vi "CreateFixedLengthString.vi"(10 "RequiredStringLength":i32, 11 "StringIn":string) -> (2 "ByteArray":u8[](array[numeric]), 3 "DLLString":string)   [LabVIEW 2023]
doc: "Use this convenience VI when providing a string of a certain length (filled with NULL) is required. Typically when writing a SDT-file.\n\ninfo@becker-hickl.com"
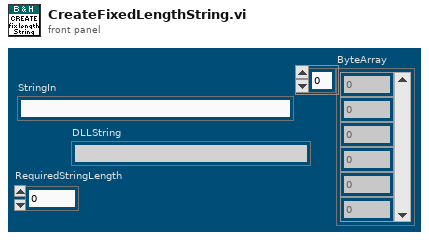
[diagram p1: front panel]
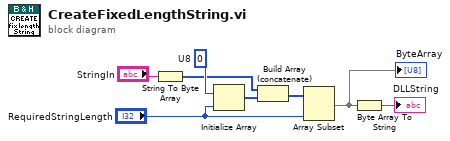
[diagram p0: block diagram]
diagram:
  w8 = u8 0  # U8
  n1 = String To Byte Array(string="StringIn") -> (unsigned byte array=w2:u8[])
  n2 = Initialize Array(w8, "RequiredStringLength") -> (w3:u8[])
  n3 = Build Array (concatenate)(w2, w3) -> (w4:u8[])
  n4 = Array Subset(array=w4, length="RequiredStringLength") -> (w6:u8[])  [unwired: 1 in]
  "ByteArray" <- w6
  n5 = Byte Array To String(unsigned byte array=w6) -> (string=→"DLLString":string)
